vi "ClearTreeNode.vi"(8 "error in":errorcluster, 10 "tag":string, 11 "tree reference":refnum<vi>) -> (0 "error out":errorcluster)   [LabVIEW 2023, in "CEF.lvlib"]
doc: "Copyright 2017 National Instruments Corporation\n\nLicensed under the Apache License, Version 2.0 (the \"License\"); you may not use this file except in compliance with the License. You may obtain a copy of the License at http://www.apache.org/licenses/LICENSE-2.0\nUnless required by applicable law or agreed to in writing, software distributed under the License is distributed on an \"AS IS\" BASIS, WITHOUT WARRANTIES OR CONDITIONS OF ANY KIND, either express or implied. See the License for the specific language governing permissions and limitations under the License."
uses:
  CEF.lvlib
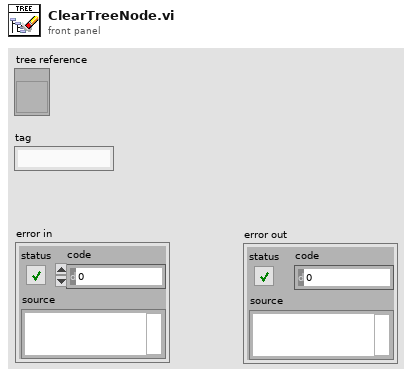
[diagram p1: front panel]
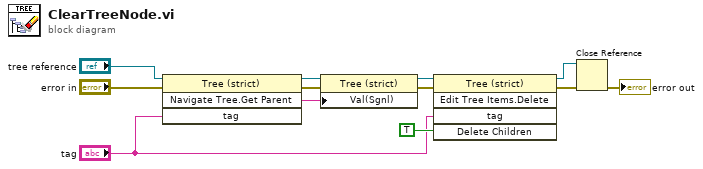
[diagram p0: block diagram]
diagram:
  n1 = invoke class="Tree (strict)" method="Navigate Tree.Get Parent"(reference="tree reference", error in="error in", "tag"="tag") -> (reference out=w8:refnum<vi>, error out=w9:errorcluster, "Navigate Tree:Get Parent"=w10:string)  [unwired: 1 in, 1 out]
  n2 = property class="Tree (strict)"(reference=w8, error in=w9, "Val(Sgnl)"=w10) -> (reference out=w12:refnum<vi>, error out=w11:errorcluster)
  n3 = invoke class="Tree (strict)" method="Edit Tree Items.Delete"(reference=w12, error in=w11, "tag"="tag", "Delete Children"=TRUE ("Delete Children?")) -> (reference out=w5:refnum<vi>, error out=w6:errorcluster)  [unwired: 1 in, 3 out]
  n4 = Close Reference(reference=w5, error in (no error)=w6) -> (error out=→"error out":errorcluster)
